vi "UA过程中等待恒温槽稳定.vi"(9 "历史数据":dbl[](array[numeric]), 10 "反应温度":dbl format="%#_13g", 11 "保温槽温度/设定温度":dbl format="%#_13g") -> (2 "三温数据":dbl[](array[numeric]), 3 "平稳":bool)   [LabVIEW 2023]
panel:
  out "求和":dbl
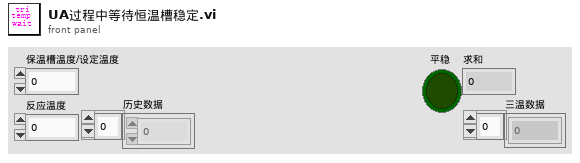
[diagram p1: front panel]
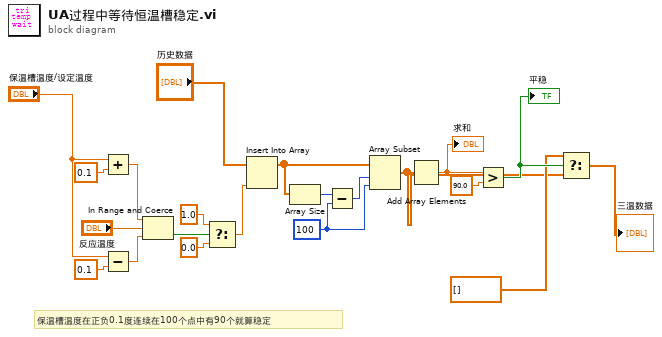
[diagram p0: block diagram]
diagram:
  w9 = 100 ("y")
  # "保温槽温度在正负0.1度连续在100个点中有90个就算稳定"
  n1 = Add(x="保温槽温度/设定温度", y=0.1) -> (x+y=w21:dbl)
  n2 = Subtract(x="保温槽温度/设定温度", y=0.1) -> (x-y=w19:dbl)
  n3 = In Range and Coerce(upper limit=w21, x="反应温度", lower limit=w19) -> (In Range?=w6:bool)  [unwired: 1 out]
  n4 = Select(t=1.0, s=w6, f=0.0) -> (s? t:f=w13:dbl)
  n5 = Insert Into Array(array="历史数据", new element=w13) -> (w12:dbl[])  [unwired: 1 in]
  n6 = Array Size(array=w12) -> (size(s)=w11:i32)
  n7 = Subtract(x=w11, y=w9) -> (x-y=w10:i32)
  n8 = Array Subset(array=w12, index=w10, length=w9) -> (w2:dbl[])
  n9 = Add Array Elements(numeric array=w2) -> (sum=w8:dbl)
  "求和" <- w8
  n10 = Greater?(x=w8, y=90.0) -> (0:w4:bool)
  "平稳" <- w4
  n11 = Select(t=dbl[] [] ("三温数据"), s=w4, f=w2) -> (s? t:f=→"三温数据":dbl[])
